vi "Unary adas_NodeCustomService_SetExample_2.vi"(8 "error in":errorcluster, 9 "timeout (ms)":i32=-1, 10 "Request Data":T2, 11 "gRPC ID":T3) -> (0 "error out":errorcluster, 2 "Response Data":T1, 3 "gRPC ID out":T3)   [LabVIEW 2019, in "Example_2_client.lvlib"]
uses:
  Example_2_client.lvlib
  RPC Messages/adas_empty.ctl
  3e2e6000-329f-4574-bb7f-38a2d219bee3.vi
  <vilib>/gRPC/LabVIEW gRPC Library/Shared/grpcId.ctl
  <vilib>/gRPC/LabVIEW gRPC Library/grpc-lvsupport-release.lvlib
  RPC Messages/adas_SetNumber.ctl
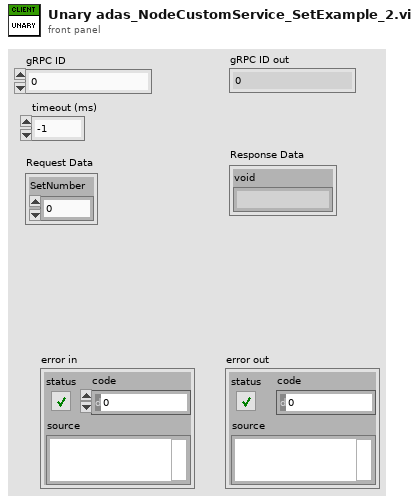
[diagram p1: front panel]
types:
  T1 = typedef "Example_2_client.lvlib/adas_empty.ctl" = cluster{"void":string}
  T2 = typedef "Example_2_client.lvlib/adas_SetNumber.ctl" = cluster{"SetNumber":u32}
  T3 = typedef "grpc-lvsupport-release.lvlib/grpcId.ctl" = u64
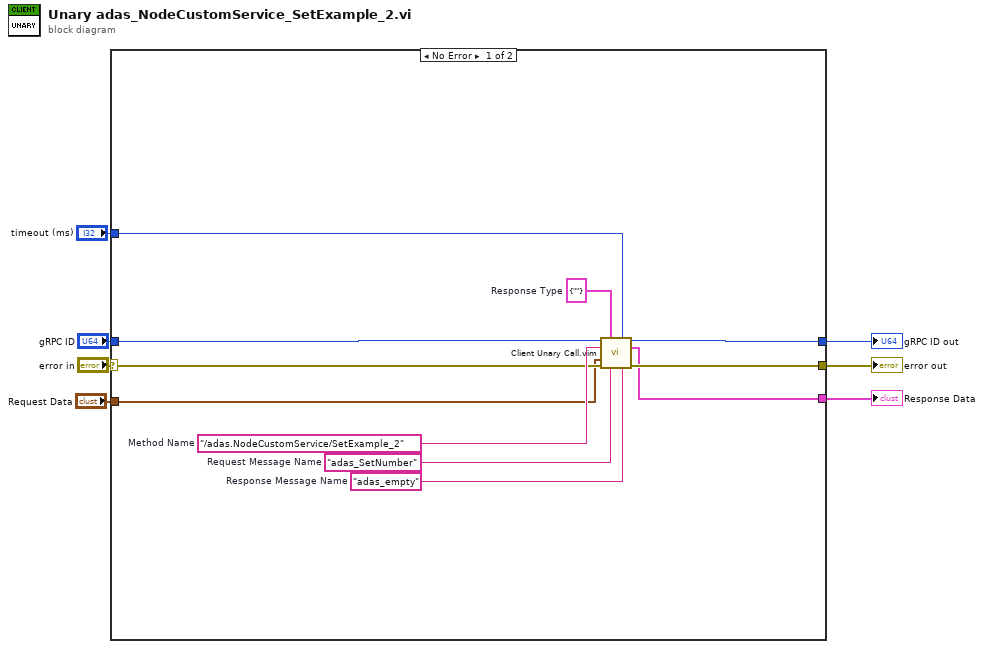
[diagram p0: block diagram]
diagram:
  n1 = case shown="No Error" "error in" {
    selector: "error in" -> [w14 w19]
    tunnel: [w13 w19] -> w6
    tunnel: "gRPC ID" -> [w12 w20]
    tunnel: [w11 w20] -> w4
    tunnel: "Request Data" -> [w10 _]
    tunnel: [w9 _] -> w2
    tunnel: "timeout (ms)" -> [w8 _]
    frame No Error {
      w15 = "adas_empty"  # Response Message Name
      w16 = "adas_SetNumber"  # Request Message Name
      w17 = T1 {"void"=""}  # Response Type
      w18 = "/adas.NodeCustomService/SetExample_2"  # Method Name
      n2 = call "Client Unary Call.vim"("ClientID in"=w12, "Response Type"=w17, "timeout (ms)"=w8, "Method Name"=w18, "Request Data"=w10, "error in"=w14, "Request Message Name"=w16, "Response Message Name"=w15) -> ("ClientID out"=w11:u64, "Response Data"=w9:T1, "error out"=w13:errorcluster)  [unwired: 5 in]
    }
    frame Error {
    }
  }
  "error out" <- w6
  "gRPC ID out" <- w4
  "Response Data" <- w2
